vi "Read Data.vi"(8 "error in (no error)":errorcluster, 10 "Read Size":i32, 11 "AcquireTraces in":refnum<class "AcquireTraces.lvclass">) -> (0 "error out":errorcluster, 2 "data":i32[][](array[numeric]), 3 "AcquireTraces out":refnum<class "AcquireTraces.lvclass">)   [LabVIEW 2014, in "AcquireTraces.lvclass"]
uses:
  AcquireTraces.lvclass
  AcquireTraces.lvclass/AcquireTraces.ctl
  <vilib>/DAQmx/read.llb/DAQmx Read (Analog 2D I32 NChan NSamp).vi
  <resource>/objmgr/daqmx.rc
panel:
  out "size(s)":i32[](array[numeric])
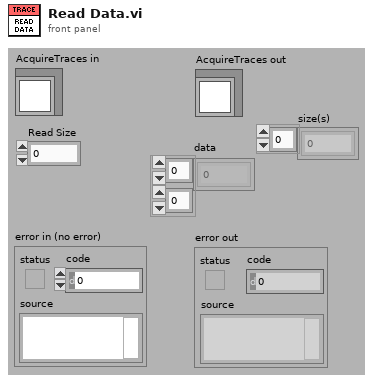
[diagram p1: front panel]
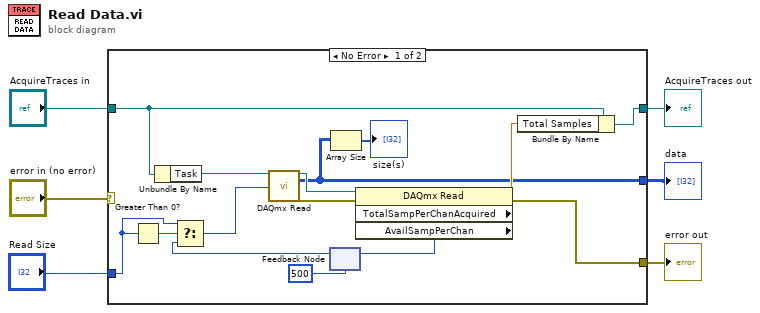
[diagram p0: block diagram]
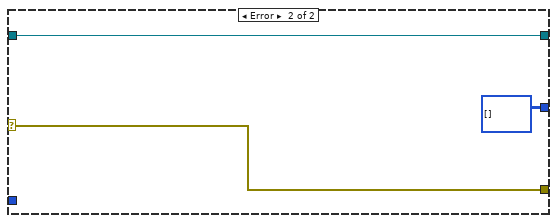
[diagram p2: hidden frame]
diagram:
  n1 = case shown="No Error" "error in (no error)" {
    selector: "error in (no error)" -> [_ w24]
    tunnel: [w16 w24] -> w5
    tunnel: [w13 w23] -> w3
    tunnel: "AcquireTraces in" -> [w14 w23]
    tunnel: [w12 i32[][] [] ("data")] -> w2
    tunnel: "Read Size" -> [w9 _]
    frame No Error {
      n2 = Greater Than 0?(x=w9) -> (x > 0?=w10:bool)
      n3 = Unbundle By Name(w14) -> ("Task"=w17:refnum<k21>)
      n4 = feedback #1(u32 500 ("AvailSampPerChan")) -> (w8:u32)
      n5 = Select(t=w9, s=w10, f=w8) -> (s? t:f=w7:u32)
      n6 = call-poly <vilib>:"DAQmx Read.vi"("task/channels in"=w17, "number of samples per channel"=w7) -> ("task out"=w21:refnum<k21>, "data"=w12:i32[][], "error out"=w18:errorcluster)  [unwired: 11 in]
      n7 = Array Size(array=w12) -> (size(s)=→"size(s)":i32[])
      n8 = property class="DAQmx Read"(reference=w21, error in=w18) -> (error out=w16:errorcluster, "TotalSampPerChanAcquired"=w15:dbl, "AvailSampPerChan"=w20:u32)  [unwired: 1 out]
      n9 = feedback-in #1(w20) -> ()
      n10 = Bundle By Name(cluster=w14, "Total Samples"=w15) -> (w13:refnum<class "AcquireTraces.lvclass">)
    }
    frame Error {
    }
  }
  "error out" <- w5
  "AcquireTraces out" <- w3
  "data" <- w2
